vi "ConvertMousePosition.vi"(0 "reference in":refnum<class "LcPictureBox.lvclass">, 2 "X":i32, 3 "Y":i32, 5 "Error In":errorcluster) -> (14 "reference out":refnum<class "LcPictureBox.lvclass">, 16 "X-Out":sgl, 17 "Y-Out":sgl, 19 "Error Out":errorcluster)   [LabVIEW 2020, in "LcPictureBox.lvclass"]
uses:
  LcPictureBox.lvclass
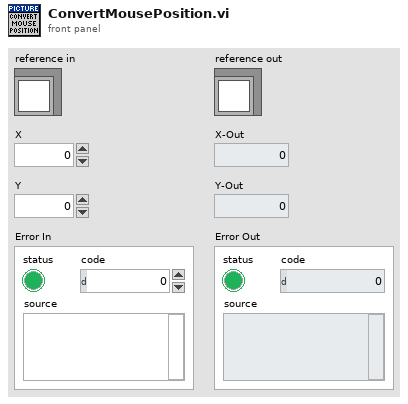
[diagram p1: front panel]
types:
  T1 = typedef "LcPictureBox.lvclass/ObjectAttributes.ctl" = cluster{"PictureBox":refnum<k24>, "ImageSize":cluster{"Width":i32, "Height":i32}, "PenMemory":map{cluster{"Alpha(100%)":dbl, "Color(Black)":u32, "Pen(Width=1, Solid)":T2}, refnum<k24>}, "GraphicsRef":refnum<k24>, "BrushMemory":map{cluster{"Alpha(100%)":dbl, "Color(Black)":u32}, refnum<k24>}, "Images":refnum<k24>[], "ImageIndex":i32, "BgColor(None)":u32, "LoadedImages":map{string, cluster{"ImageOut":refnum<k24>, "ImageSize":cluster{"Width":i32, "Height":i32}}}, "ColorsMemory":map{cluster{"Alpha(100%)":dbl, "Color(Black)":u32}, refnum<k24>}, "CacheSize":i32, "PictureBoxActiveXReference":refnum<vi>, "Scale":dbl, "Offset":cluster{"x":sgl, "y":sgl}, "zoom_center":cluster{"X":i32, "Y":i32}, "ImagesCreated":refnum<k24>[], "CustomCursorImages":map{u16, refnum<k24>}}
  T2 = typedef "LcPictureBox.lvclass/Pen.ctl" = cluster{"Width":u16, "Style":enum32{"Solid", "Dash", "Dot", "DashDot", "DashDotDot"}}
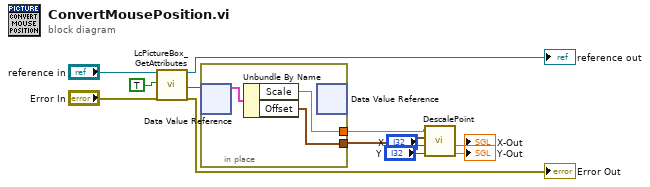
[diagram p0: block diagram]
diagram:
  n1 = call "LcPictureBox_GetAttributes.vi"("reference in"="reference in", "OnlyGetDvrReference(False)"=TRUE, "error in (no error)"="Error In") -> ("reference out"=→"reference out":refnum<class "LcPictureBox.lvclass">, "DataRef"=w8:refnum<data-value>, "error out"=→"Error Out":errorcluster)  [unwired: 13 in, 1 out]
  n2 = in-place {
    in-place-border: [w14] -> w5
    in-place-border: [w13] -> w6
    n3 = in-place-dvr #1(w8) -> (w15:T1)  [unwired: 1 out]
    n4 = Unbundle By Name(w15) -> ("Scale"=w13:dbl, "Offset"=w14:cluster{"x":sgl, "y":sgl})
    n5 = in-place-dvr #1() -> ()  [unwired: 1 in, 2 out]
  }
  n6 = call "DescalePoint.vi"("Y"="Y", "X"="X", "Offset"=w5, "Scale"=w6) -> ("Y-Out"=→"Y-Out":sgl, "X-Out"=→"X-Out":sgl)  [unwired: 6 in]
